vi "TestExec.Set Child Application Window State.vi"(1 "This VI":refnum<vi>) -> (0 "TE Running":bool)   [LabVIEW 2019]
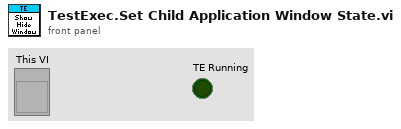
[diagram p1: front panel]
types:
  T1 = enum32{"invalid app kind", "Development System", "Run Time System", "Student Edition", "Embedded LabVIEW", "Evaluation", "Custom"}
  T2 = enum32{"Invalid", "Standard", "Closed", "Hidden", "Minimized", "Maximized"}
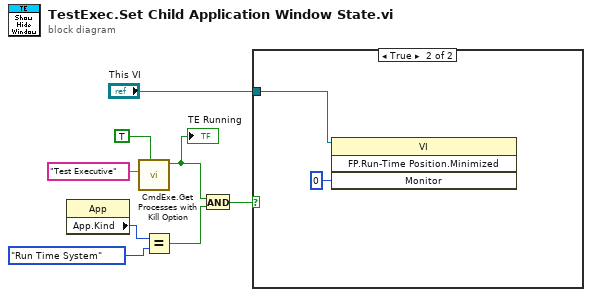
[diagram p0: block diagram]
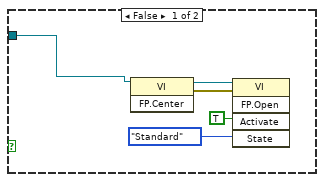
[diagram p2: hidden frame]
diagram:
  n1 = property class="App"() -> ("App.Kind"=w6:T1)  [unwired: 2 in, 2 out]
  n2 = call "CmdExe.Get Processes with Kill Option.vi"("Name Contains"=TRUE, "Process Name"="Test Executive") -> ("Is Running"=w2:bool)  [unwired: 6 in, 3 out]
  "TE Running" <- w2
  n3 = Equal?(x=w6, y=T1."Run Time System" ("Application:Kind")) -> (x = y?=w4:bool)
  n4 = And(x=w2, y=w4) -> (x .and. y?=w3:bool)
  n5 = case shown="True" w3 {
    tunnel: "This VI" -> [w9 w15]
    frame False {
      n6 = invoke class="VI" method="FP.Center"(reference=w9) -> (reference out=w12:refnum<vi>, error out=w13:errorcluster)  [unwired: 2 in, 1 out]
      n7 = invoke class="VI" method="FP.Open"(reference=w12, error in=w13, "Activate"=TRUE ("Activate?"), "State"=T2."Standard") -> ()  [unwired: 1 in, 5 out]
    }
    frame True {
      n8 = invoke class="VI" method="FP.Run-Time Position.Minimized"(reference=w15, "Monitor"=i16 0) -> ()  [unwired: 2 in, 4 out]
    }
  }
